vi "LSL with LVCS.vi"() -> ()   [LabVIEW 2016]
uses:
  source code/LSL components/output terminal/Plain OT/PainOutputTerminal.lvclass
  E:/Repository/LabVIEW Script Language/source code/LSL components/output terminal/Base/Output Terminal.lvclass
  source code/LSL components/scripts/scripts manager/scripts manager.lvclass
  source code/LSL components/variables/RT Variables/RT Variables.lvclass
  source code/LSL components/output terminal/Plain OT/PainOutputTerminal.lvclass/PainOutputTerminal.ctl
  <vilib>/ADI/Code String/Code String/Code String/Code String__adi.lvclass/Code String__adi.ctl
  source code/LSL components/scripts/scripts manager/scripts manager.lvclass/scripts manager.ctl
  source code/LSL components/scripts/scripts manager/properties/Write Scripts.vi
  source code/LSL components/output terminal/Plain OT/properties/Write Output Terminal.vi
  <vilib>/ADI/Code String/Code String/Code String LV/Code String LV__adi.lvclass
  C:/Program Files (x86)/National Instruments/LabVIEW 2016/vi.lib/ADI/Code String/Code String/Code String/Code String__adi.lvclass
  <vilib>/ADI/Code String/Code String/Code String LV/Create Code String LV.vi
  source code/LSL components/scripts/scripts manager/properties/Get Keywords.vi
  <vilib>/ADI/Code String/Code String/Code String/Properties/Write Keywords.vi
  <vilib>/ADI/Code String/Code String/Code String/Properties/Write Font Size.vi
  <vilib>/ADI/Code String/Code String/Code String/Properties/Write Completion.vi
  <vilib>/ADI/Code String/Code String/Code String/Properties/Write Delimiter Pattern.vi
  <vilib>/ADI/Code String/Code String/Code String/Properties/Write Editable.vi
  <vilib>/ADI/Code String/Code String/Code String/Properties/Write Text.vi
  <vilib>/ADI/Code String/Code String/Code String/Properties/Write Scroll Position.vi
  <vilib>/ADI/Code String/Code String/Code String/Properties/Write Selected Text.vi
  <vilib>/ADI/Code String/Code String/Code String/Properties/Write Font Color.vi
  <vilib>/ADI/Code String/Code String/Code String/Properties/Write Selection End.vi
  <vilib>/ADI/Code String/Code String/Code String/Properties/Write Selection Start.vi
  <vilib>/ADI/Code String/Code String/Code String/Properties/Read Selected Line(s).vi
  <vilib>/ADI/Code String/Code String/Code String/Properties/Read Selected Token.vi
  <vilib>/ADI/Code String/Code String/Code String/Properties/Read # Selected Lines.vi
  <vilib>/ADI/Code String/Code String/Code String/Properties/Read Selected Text.vi
  <vilib>/ADI/Code String/Code String/Code String/Properties/Read Text.vi
  <vilib>/ADI/Code String/Code String/Code String/Code String__adi.lvclass
panel:
  in  "Script Run":bool
  out "Output Terminal":string
  in  "Replacement Text":string="Test"
  in  "Replace Selection":bool
  out "Selected Text":string
  out "# Lines":i32
  out "Selected Token":string
  out "Selected Line(s)":string
  in  "Auto-complete":bool=TRUE
  in  "Editable":bool=TRUE
  in  "Checked?":bool
  out "Selected Menu Item":string
  in  "Item Name/Tag":string
  in  "Visible?":bool
  in  "Set Menu Item":bool
  in  "Selection End":u32
  in  "Selection Start":u32
  in  "Font Color":u32(colorbox)
  in  "Add Text":bool
  in  "Font Size":u32=14
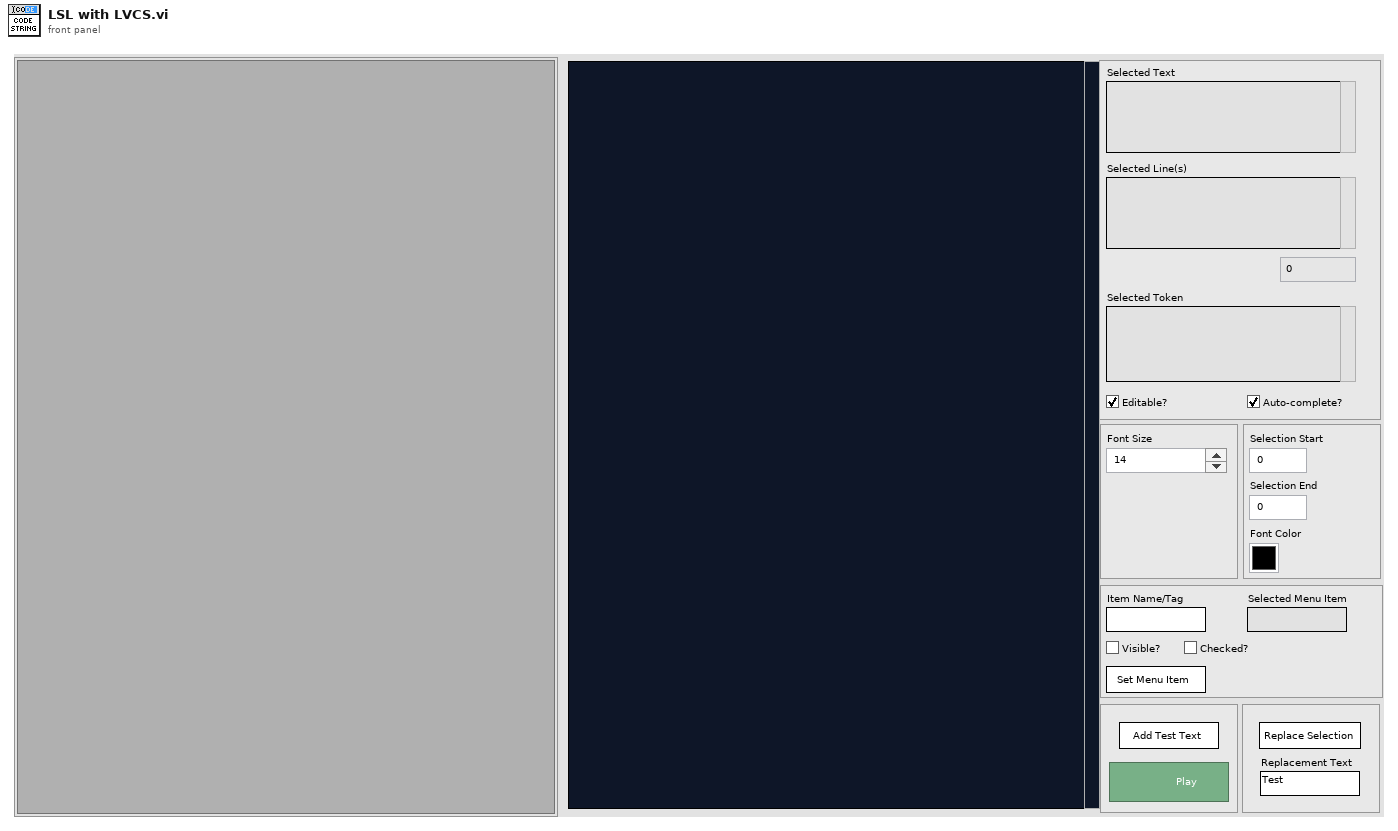
[diagram p1: front panel]
types:
  T1 = typedef "Code String__adi.lvclass/Public Events.ctl" = cluster{"Selected Token Changed":refnum<user-event>, "Value Changed":refnum<user-event>, "Shortcut Menu Selection":refnum<user-event>}
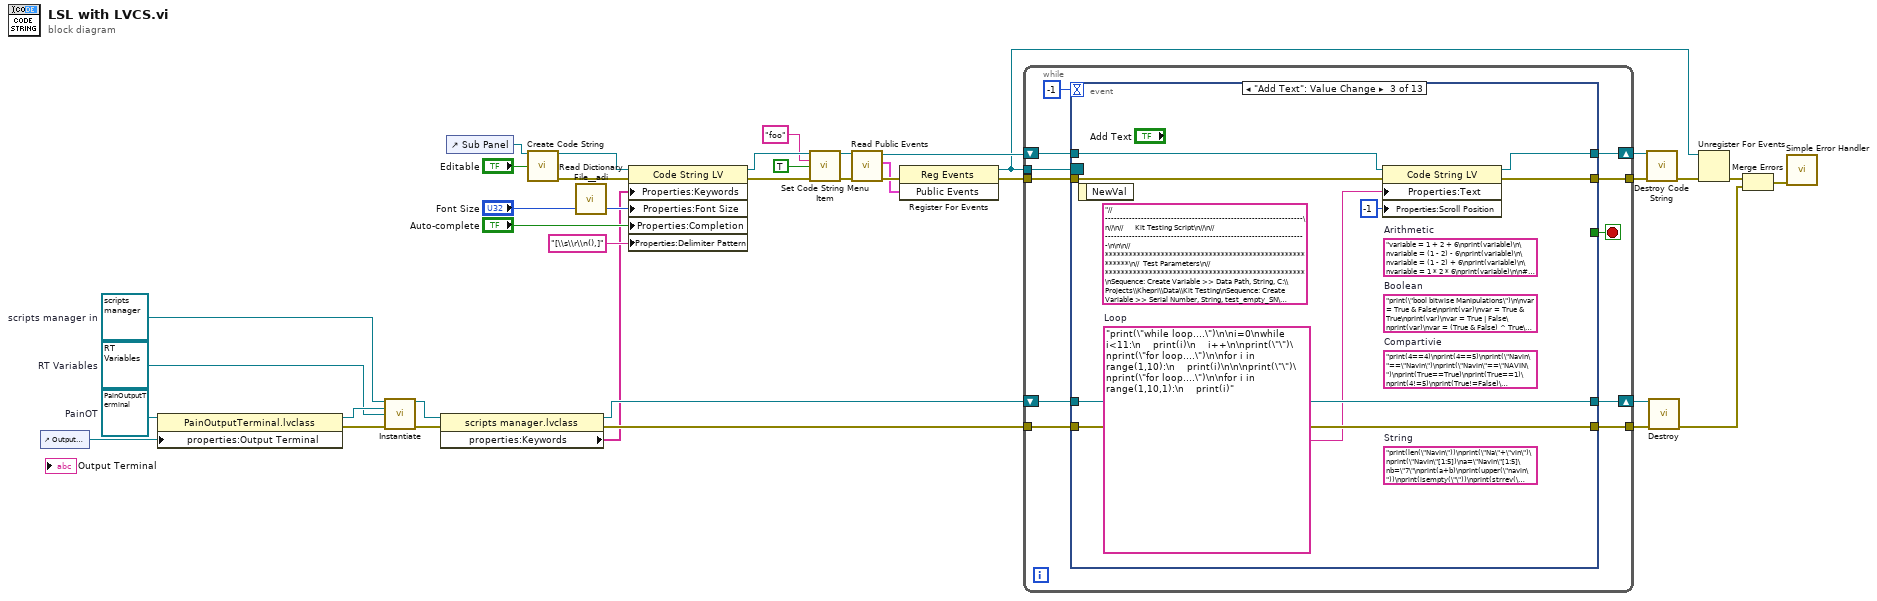
[diagram p0: block diagram]
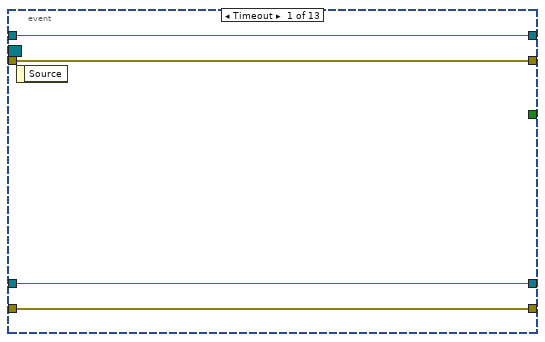
[diagram p2: hidden frame]
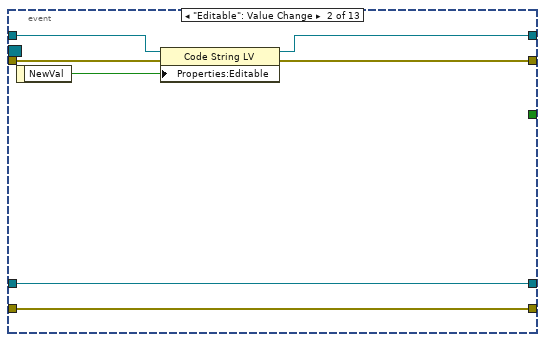
[diagram p3: hidden frame]
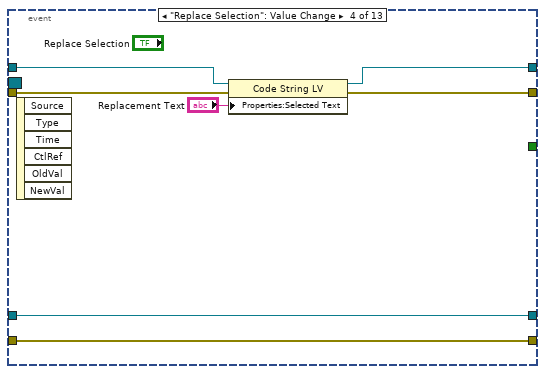
[diagram p4: hidden frame]
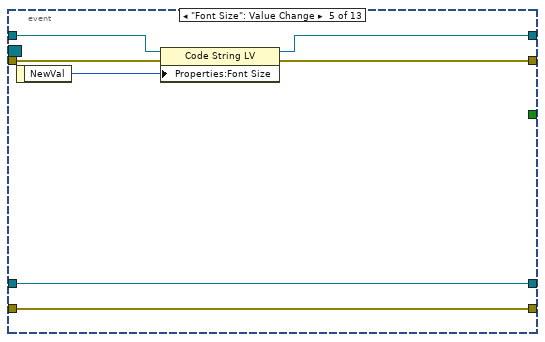
[diagram p5: hidden frame]
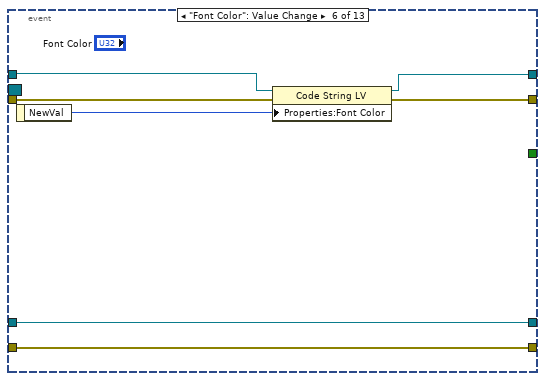
[diagram p6: hidden frame]
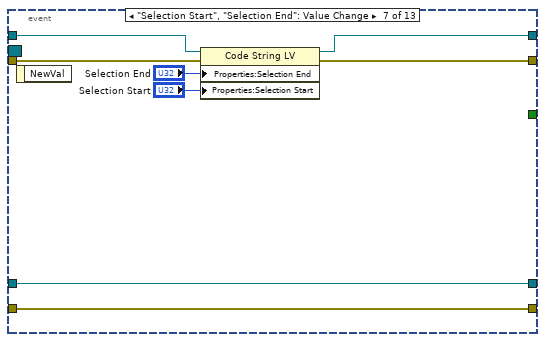
[diagram p7: hidden frame]
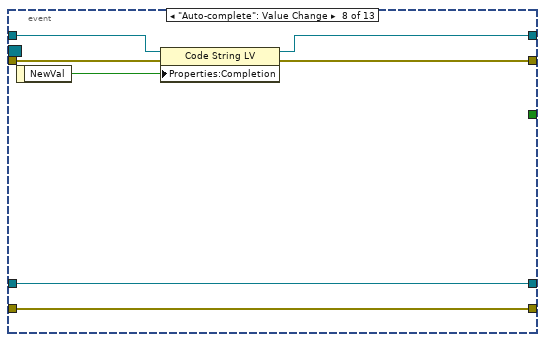
[diagram p8: hidden frame]
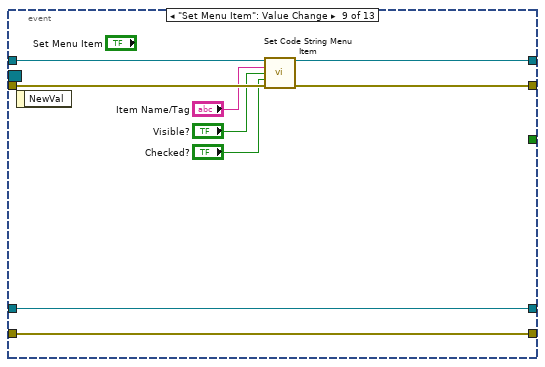
[diagram p9: hidden frame]
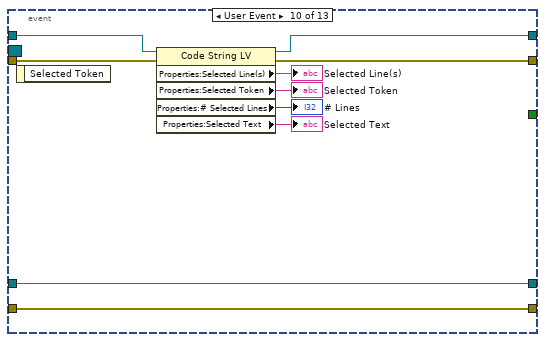
[diagram p10: hidden frame]
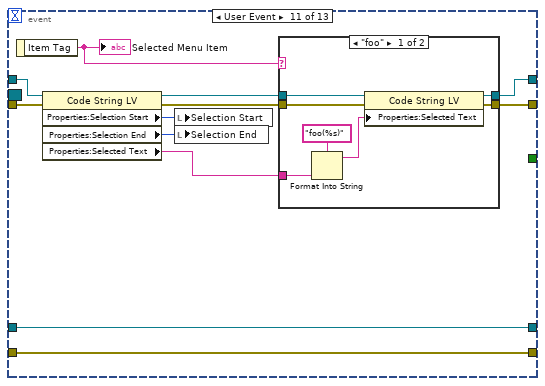
[diagram p11: hidden frame]
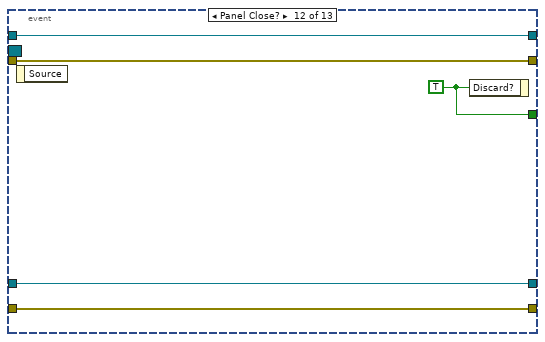
[diagram p13: hidden frame]
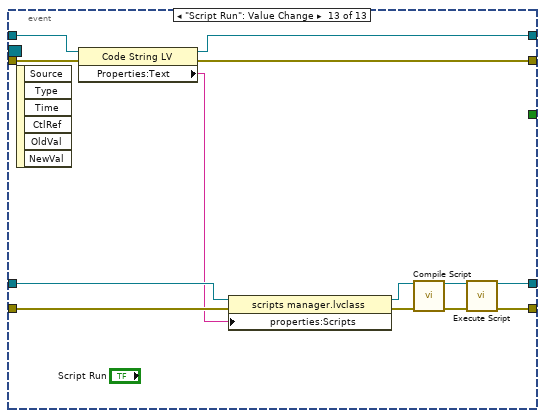
[diagram p14: hidden frame]
diagram:
  w10 = refnum<class "RT Variables.lvclass"> refnum  # RT Variables
  w12 = refnum<class "scripts manager.lvclass"> refnum  # scripts manager in
  w15 = refnum<class "PainOutputTerminal.lvclass"> refnum  # PainOT
  n1 = control-ref of="Output Terminal"() -> (w14:refnum<vi>)
  n2 = property class="PainOutputTerminal.lvclass"(reference=w15, "properties:Output Terminal"=w14) -> (reference out=w11:refnum<class "PainOutputTerminal.lvclass">, error out=w13:errorcluster)  [unwired: 1 in]
  n3 = call-dynamic "Instantiate.vi"("scripts manager in"=w12, "Output Terminal"=w11, "RT Variables"=w10, "error in (no error)"=w13) -> ("scripts manager out"=w3:refnum<class "scripts manager.lvclass">, "error out"=w9:errorcluster)  [unwired: 10 in]
  n4 = property class="scripts manager.lvclass"(reference=w3, error in=w9) -> (reference out=w2:refnum<class "scripts manager.lvclass">, error out=w4:errorcluster, "properties:Keywords"=w1:string[])
  n5 = control-ref of="Sub Panel"() -> (w21:refnum<vi>)
  n6 = call-poly <vilib>:"Create Code String.vi"("Subpanel"=w21, "Editable? (T)"="Editable") -> ("Code String LV"=w37:refnum<class "Code String LV__adi.lvclass">, "error out"=w33:errorcluster)  [unwired: 12 in]
  n7 = call "Read Dictionary File__adi.vi"() -> ()  [unwired: 3 in, 1 out]
  n8 = property class="Code String LV"(reference=w37, error in=w33, "Properties:Keywords"=w1, "Properties:Font Size"="Font Size", "Properties:Completion"="Auto-complete", "Properties:Delimiter Pattern"="[\\s\\r\\n(),]") -> (reference out=w19:refnum<class "Code String LV__adi.lvclass">, error out=w32:errorcluster)
  n9 = call <vilib>:"Set Code String Menu Item.vi"("Code String in"=w19, "Item Path"="foo", "Visibility (T)"=TRUE, "error in (no error)"=w32) -> ("Code String out"=w18:refnum<class "Code String LV__adi.lvclass">, "error out"=w20:errorcluster)  [unwired: 10 in]
  n10 = call <vilib>:"Read Public Events.vi"("error in (no error)"=w20, "Code String in"=w18) -> ("error out"=w29:errorcluster, "Public Events"=w26:T1, "Code String out"=w28:refnum<class "Code String LV__adi.lvclass">)  [unwired: 7 in]
  n11 = register-events(error in=w29, w26) -> (reference out=w23:refnum<event-registration>, error out=w27:errorcluster)  [unwired: 1 in]
  n12 = while {
    shift-right: [w47] -> w36
    shift-left: w28 -> [w48]
    tunnel: w27 -> [w46]
    tunnel: [w45] -> w35
    tunnel: w23 -> [w42]
    shift-right: [w39] -> w8
    shift-left: w2 -> [w41]
    tunnel: w4 -> [w40]
    tunnel: [w38] -> w7
    stop <- w43 stop-if-true
    n13 = event shown="[2] \"Add Text\": Value Change" {
      selector: w42 -> [_ _ _ _ _ _ _ _ _ _ _ _ _]
      dyn-events: _ -> [_ _ _ _ _ _ _ _ _ _ _ _ _]
      timeout: -1 -> [_ _ _ _ _ _ _ _ _ _ _ _ _]
      tunnel: w48 -> [w52 w58 w66 w72 w79 w84 w94 w101 w110 w120 w133 w146 w151]
      tunnel: [w52 w57 w65 w71 w78 w86 w93 w100 w109 w119 w126 w146 w150] -> w47
      tunnel: w46 -> [w51 w59 w67 w74 w81 w88 w96 w103 w112 w118 w134 w147 w153]
      tunnel: [w51 w56 w63 w73 w80 w87 w95 w102 w111 w117 w125 w147 w152] -> w45
      tunnel: [_ _ _ _ _ _ _ _ _ _ _ w148 _] -> w43
      tunnel: w41 -> [w50 w54 w62 w69 w76 w83 w90 w98 w105 w114 w124 w145 w159]
      tunnel: w40 -> [w49 w53 w61 w68 w75 w82 w89 w97 w104 w113 w123 w144 w161]
      tunnel: [w50 w54 w62 w69 w76 w83 w90 w98 w105 w114 w124 w145 w154] -> w39
      tunnel: [w49 w53 w61 w68 w75 w82 w89 w97 w104 w113 w123 w144 w155] -> w38
      event Timeout {
        n14 = event-data() -> ()  [unwired: 1 in, 1 out]
      }
      event "Editable": Value Change {
        n15 = event-data() -> ("NewVal"=w55:bool)  [unwired: 1 in]
        n16 = property class="Code String LV"(reference=w58, error in=w59, "Properties:Editable"=w55) -> (reference out=w57:refnum<class "Code String LV__adi.lvclass">, error out=w56:errorcluster)
      }
      event "Add Text": Value Change {
        (unwired) "print(len(\"Navin\"))\nprint(\"Na\"+\"vin\")\nprint(\"Navin\"[1:5])\na=\"Navin\"[1:5]\nb=\"7\"\nprint(a+b)\nprint(upper(\"navin\"))\nprint(isempty(\"\"))\nprint(strrev(\"navin\"))\n\na = \"Hello World!!!\"\nprint(a[1:6])\nprint(a[6])\n"  # String
        w60 = "print(\"while loop....\")\n\ni=0\nwhile i<11:\n    print(i)\n    i++\n\nprint(\"\")\nprint(\"for loop....\")\n\nfor i in range(1,10):\n    print(i)\n\n\nprint(\"\")\nprint(\"for loop....\")\n\nfor i in range(1,10,1):\n    print(i)"  # Loop
        (unwired) "print(4==4)\nprint(4==5)\nprint(\"Navin\"==\"Navin\")\nprint(\"Navin\"==\"NAVIN\")\nprint(True==True)\nprint(True==1)\nprint(4!=5)\nprint(True!=False)\nprint(1>2)\nprint(1<2)\nprint(1>=2)\nprint(1<=2)\n"  # Compartivie
        (unwired) "print(\"bool bitwise Manipulations\")\n\nvar = True & False\nprint(var)\nvar = True & True\nprint(var)\nvar = True | False\nprint(var)\nvar = (True & False) ^ True\nprint(var)\n\nprint(\"\")\nprint(\"numeric bitwise Manipulations\")\n\nvar1 = 1\nvar2 = 2\nprint(var1 & var2)\nprint(var1 | var2)\nprint(var1 ^ var2)\n\nprint(\"\")\nprint(\"bool Manipulations\")\n\nvar = True and False\nprint(var)\nvar = True and True\nprint(var)\nvar = True or False\nprint(var)\nvar = (True and False) xor True\nprint(var)\nprint(not(var))\n\nprint(\"\")\nprint(\"other functions\")\n\nprint(randombool())"  # Boolean
        (unwired) "variable = 1 + 2 + 6\nprint(variable)\n\nvariable = (1 - 2) - 6\nprint(variable)\n\nvariable = (1 - 2) + 6\nprint(variable)\n\nvariable = 1 * 2 * 6\nprint(variable)\n\n# a = gettick()\n\n#variable = (1 - 2) - (7-8) + (7/3.5) * 5 + (5+5) / 6 * 2 -1\nprint(variable)\n\n# print(\"time taken is : \"+str((gettick()-a)))\n\n# print(randomnumber())\n\n#the operation works from right to left\nvariable = (1 / 2 )/ 6\nprint(variable)\n\n#combination of operation\n\nvariable = 1 + 2 * 6 / 2\nprint(variable)\n\nvariable = 1 / 2 * 6 / 2\nprint(variable)\n\nvariable = 1 / 2 + 6 / 2\nprint(variable)\n\nvariable = ((1 / 2) - (6 * 2)) + 6.5\nprint(variable)\n\n# i=0\n# print(i++)\n# print(i--)\n\nvariable = ((1 - 2) - (6 * 2)) + 6.5\nprint(variable)\n\nvariable = 4%3\nprint(variable)\nprint(4%4)\nprint(4%5)\nprint(4%2)\n\nprint(4**2)\n\nprint(4//2)"  # Arithmetic
        (unwired) "//------------------------------------------------------------------\n//\n//      Kit Testing Script\n//\n//-------------------------------------------------------------------\n\n\n//********************************************************\n//  Test Parameters\n//**************************************************\nSequence: Create Variable >> Data Path, String, C:\\Projects\\Khepri\\Data\\Kit Testing\nSequence: Create Variable >> Serial Number, String, test_empty_SN\nSequence: Create Variable >> Noise Views, Integer, 512\n\nKit Testing: Scan Serial Number\nSequence: Update Variable >> Serial Number, = %Scanned Serial Number%\n\n//********************************************************\n// Sequence Variables\n//********************************************************\nSequence: Create Variable >> Gain, Integer, 0\nSequence: Create Variable >> Channel Counter, Integer, 0\n\n\n//Create a data folder for the serial number\nKit Testing: Create Folder >> %Data Path%\\%Serial Number%\nReports: Set Report Path >> %Data Path%\\%Serial Number%\n\n\nSequence: Library Call >> Board Control Library, Initialize Eval Boards\nDS: Write Value >> Eval_Register_Map/EvalRegMap:IO_CONTROL:IO_BGN_CTRL, = 0\nControl: Update Control Value >> View Rate, = 10\nControl: Update Control Value >> View Rate Slider, = 50\nControl: Update Control Value >> Set View Rate, = 1, Trigger\nSequence: Library Call >> Linearity Library, Clear 18bit Mode\n\n//%%%%%%%%%%%%%%%%%%%%%%%%%%%%%%%%%%%%%%%%%%%%%%%%%%\n//  Power Measurements\n//%%%%%%%%%%%%%%%%%%%%%%%%%%%%%%%%%%%%%%%%%%%%%%%%%%\n\nReports: New Datalog >> Voltage, Current\nPanels: Send Sync Command >> PXI-4113 - 1, 500, UI: Front Panel State >> Open\nPanels: Send Sync Command >> PXI-4113 - 2, 500, UI: Front Panel State >> Open\n\nPanels: Send Sync Command >>PXI-4113 - 1, 2000, Control: Update Control Value >> PXI 4113 Panel.CH0 Output, = 1, Trigger\nPanels: Send Sync Command >>PXI-4113 - 1, 2000, Control: Update Control Value >> PXI 4113 Panel.CH1 Output, = 1, Trigger\nPanels: Send Sync Command >>PXI-4113 - 2, 2000, Control: Update Control Value >> PXI 4113 Panel.CH1 Output, = 1, Trigger\nPanels: Send Sync Command >>PXI-4113 - 2, 2000, Control: Update Control Value >> PXI 4113 Panel.CH0 Output, = 1, Trigger\n\nUI: Generate Popup >> Move switch away from FPGA (LED off), then close shield\nDS: Write Value >> Eval_Register_Map/EvalRegMap:RELAYS_5:HB2, = 0\nFunction: Wait >> 0.1\nDS: Write Value >> Eval_Register_Map/EvalRegMap:RELAYS_5:HB2, = 1\nExperiments: Program FPGA >> C:\\Projects\\Khepri\\Labview\\Firmware\\Sphinx\\sphinx_320ADC_DBG_051818.bin\n\n//Wait 5 seconds for the DUT board to initialize and program\nFunction: Wait >> 5\n\nPanels: Send Sync Command >>PXI-4113 - 1, 2000, Control: Update Control Value >> PXI 4113 Panel.Measure Supplies, = 1, Trigger\nPanels: Send Sync Command >>PXI-4113 - 2, 2000, Control: Update Control Value >> PXI 4113 Panel.Measure Supplies, = 1, Trigger\n\nReports: Datalog >> %PXI-4113 - 1: PXI 4113 Panel.CH0 Voltage%, %PXI-4113 - 1: PXI 4113 Panel.CH0 Current%, M{%PXI-4113 - 1: PXI 4113 Panel.CH0 Voltage% * %PXI-4113 - 1: PXI 4113 Panel.CH0 Current%}, W, Fractional, Total Power\nReports: Datalog >> %PXI-4113 - 1: PXI 4113 Panel.CH1 Voltage%, %PXI-4113 - 1: PXI 4113 Panel.CH1 Current%, M{%PXI-4113 - 1: PXI 4113 Panel.CH1 Voltage% * %PXI-4113 - 1: PXI 4113 Panel.CH1 Current%}, W, Fractional, Total Power\nReports: Datalog >> %PXI-4113 - 2: PXI 4113 Panel.CH0 Voltage%, %PXI-4113 - 2: PXI 4113 Panel.CH0 Current%, M{%PXI-4113 - 2: PXI 4113 Panel.CH0 Voltage% * %PXI-4113 - 2: PXI 4113 Panel.CH0 Current%}, W, Fractional, Total Power\nReports: Datalog >> %PXI-4113 - 2: PXI 4113 Panel.CH1 Voltage%, %PXI-4113 - 2: PXI 4113 Panel.CH1 Current%, M{%PXI-4113 - 2: PXI 4113 Panel.CH1 Voltage% * %PXI-4113 - 2: PXI 4113 Panel.CH1 Current%}, W, Fractional, Total Power \n\nReports: Set Report Name >> %Serial Number%_Power\nReports: Save Datalog >> Close\n\nPanels: Send Sync Command >> PXI-4113 - 1, 500, UI: Front Panel State >> Close\nPanels: Send Sync Command >> PXI-4113 - 2, 500, UI: Front Panel State >> Close\n\n\n//+++++++++++++++++++++++++++++++++++++++++++++++++++++++++++++++++\n//  Noise and Offset tests\n//+++++++++++++++++++++++++++++++++++++++++++++++++++++++++++++++++\nReports: New Report\n\nControl: Update Control Value >> Eval Tabs, = 0\nReports: New Datalog >> View Rate, VR Jitter, Gain, Max Offset, Min Offset, Max Noise, Mean Noise\n\n//Connect Q_BOARD_AGND_PDA to BOARD_DGND\nSequence: Library Call >> Board Control Library, Power Up Slave Eval\nSequence: Library Call >> Noise and Offset Library, Set Noise Master Relays\n//Sequence: Library Call >> Board Control Library, Power Down Slave Eval\nSequence: Call >> Initialize Noise Test Parameters\n\n\n\n//Set View rate to 3000min\nControl: Update Control Value >> View Rate, = 10\nControl: Update Control Value >> View Rate Slider, = 0\nControl: Update Control Value >> Set View Rate, = 1, Trigger\n\n//Run Noise and Offset versus gain setting\nSequence: Call >> Noise and Offset versus Gain\n\n//Set View rate to 800max\nControl: Update Control Value >> View Rate, = 0\nControl: Update Control Value >> View Rate Slider, = 100\nControl: Update Control Value >> Set View Rate, = 1, Trigger\n\n//Run Noise and Offset versus gain setting\nSequence: Call >> Noise and Offset versus Gain\n\n//Set View rate to 3000nom\nControl: Update Control Value >> View Rate, = 10\nControl: Update Control Value >> View Rate Slider, = 50\nControl: Update Control Value >> Set View Rate, = 1, Trigger\n\nReports: Set Report Name >> %Serial Number%_Noise_and_Offset\nReports: Save Datalog >> Close\n\nSequence: Library Call >> Board Control Library, Power Up Slave Eval\nSequence: Library Call >> Noise and Offset Library, Clear Noise Master Relays\n\n\n//End Noise and Offset Tests\n//+++++++++++++++++++++++++++++++++++++++++++++++++++++++++++++\n\n\n//====================================================\n//  Linearity Tests\n//====================================================\n\nReports: New Line\nControl: Update Control Value >> Eval Tabs, = 1\n\nSequence: Library Call >> Board Control Library, Power Up Slave Eval\n\nSequence: Library Call >> Board Control Library, Power Up Master Q Board\nSequence: Library Call >> Board Control Library, Power Up Slave Q Board\nFunction: Wait >> 3\n\n//Set the Analog Input Relays to connect Q board to DUT\nPanels: Send Sync Command >>Khepri Panel, 8000, Control: Update Control Value >> Set Master Analog Relays, = 1, Trigger\nPanels: Send Sync Command >>Khepri Panel, 8000, Control: Update Control Value >> Set Slave Analog Relays, = 1, Trigger\n\nSequence: Library Call >> Linearity Library, Default Linearity Processing Settings\n\n\nSequence: Library Call >> Linearity Library, Set 18bit Mode\n\n\n\nSequence: For >> Gain = 1; Gain <= 7; Gain + 1\nReports: New Datalog >> Gain, Max INL, Max INL CH, Min INL, Min INL CH, Max Gain, Max Gain CH, Min Gain, Min Gain CH\n\nDS: Write Value >> Eval_Register_Map/EvalRegMap:TRS_HEADER_DAT:GAIN, = %Gain%\nSequence: Library Call >> Linearity Library, Linearity Gain%Gain% Settings\nControl: Update Control Value >> Run Linearity, = T, Trigger\nReports: Add Comment >> Gain %Gain% Linearity\nReports: Add Picture >> Linearity\nReports: Add Picture >> Raw Data\nReports: New Page\n\nReports: Datalog >> %Gain%, %Linearity Results.Max INL%, %Linearity Results.Max INL CH%, %Linearity Results.Min INL%, %Linearity Results.Min INL CH%, %Linearity Results.Max Gain%, %Linearity Results.Max Gain CH%, %Linearity Results.Min Gain%, %Linearity Results.Min Gain CH%, 0, Linearity, Fractional, All the linearity datas\n\n\nReports: Datalog Array >> Gain per Channel, Gain per channel\nReports: Datalog Array >> DAC Input Values, Linearity Input Values\n\nSequence: For >> Channel Counter = 0; Channel Counter <= 191; Channel Counter + 1\nKit Testing: Get Linearity Ain Data >> %Channel Counter%\nReports: Datalog Array >> CH%Channel Counter% Linearity, Linearity Ain Data\nSequence: END FOR\n\nReports: Set Report Name >> %Serial Number%_G%Gain%_Linearity_and_Gain\nReports: Save Datalog >> Close\n\nSequence: END FOR\n\n\n//Open Analog Input relays again\nPanels: Send Sync Command >>Khepri Panel, 8000, Control: Update Control Value >> Reset Master Analog Relays, = 1, Trigger\nPanels: Send Sync Command >>Khepri Panel, 8000, Control: Update Control Value >> Reset Slave Analog Relays, = 1, Trigger\n\nSequence: Library Call >> Linearity Library, Clear 18bit Mode\nSequence: Library Call >> Board Control Library, Power Down Slave Q Board\nSequence: Library Call >> Board Control Library, Power Down Master Q Board\nSequence: Library Call >> Board Control Library, Power Down Slave Eval\n\n\n//End Linearity Tests\n//====================================================================\n\n\n\n//#############################################################################\n//  Input Leakage and Offset Drift\n//#############################################################################\nControl: Update Control Value >> Eval Tabs, = 4\nControl: Update Control Value >> Tests Subtabs, = 3\n\n\nReports: New Datalog >> Offset Drift\n\n//Offset drift settings\nControl: Update Control Value >> Total Time (sec), = 65\nControl: Update Control Value >> Moving Average Window, = 144\nDS: Write Value >> Eval_Register_Map/EvalRegMap:TRS_HEADER_DAT:GAIN, = 3\nDS: Write Value >> Eval_Register_Map/EvalRegMap:NUM_VIEWS_CAPT:NUM_VIEWS_CAPT, = 256\nControl: Update Control Value >> View Rate Slider, = 50\nControl: Update Control Value >> View Rate, = 10\nControl: Update Control Value >> Set View Rate, = 1, Trigger\nControl: Update Control Value >> Offset Drift Processing.Display, = 0\n\nControl: Update Control Value >> Run Offset Drift, = 1, Trigger\n\nReports: Add Picture >> Offset Drift Graph\nReports: Datalog Array >> Offset Drift, Drift Data per Channel\nReports: Set Report Name >> %Serial Number%_G3_Offset_Drift\nReports: Save Datalog >> Close\nFunction: Wait >> 2\n\n\n//This is the recorded macro sequence\n***\nReports: New Datalog >> Input Leakage\n\n//Input Leakage settings\nControl: Update Control Value >> First Edge Clock, = 775\nControl: Update Control Value >> Start Clock, = 5000\nControl: Update Control Value >> End Clock, = 12000\nControl: Update Control Value >> Num Leakage Steps, = 10\nDS: Write Value >> Eval_Register_Map/EvalRegMap:TRS_HEADER_DAT:GAIN, = 1\nDS: Write Value >> Eval_Register_Map/EvalRegMap:NUM_VIEWS_CAPT:NUM_VIEWS_CAPT, = 64\nDS: Write Value >> Eval_Register_Map/EvalRegMap:VT_LOW_BITS:VT_PERIOD, = 1000000\n\nControl: Update Control Value >> Run Input Leakage, = 1, Trigger\n\n\nReports: Datalog Array >> Input Leakage, Leakage Data per Channel\nReports: Set Report Name >> %Serial Number%_G1_Input_Leakage\nReports: Save Datalog >> Close\n***\n\nReports: Set Report Name >> %Serial Number%_Results\nReports: Save Report >> Close\n\n\nUI: Generate Popup >> Move switch toward FPGA (LED on)\nExperiments: Program EEPROM >> C:\\Projects\\Khepri\\Labview\\Firmware\\Sphinx\\sphinx_320ADC_DBG_051818.bin\n\n//Power down the board at the end of the sequence\nPanels: Send Sync Command >>PXI-4113 - 2, 2000, Control: Update Control Value >> PXI 4113 Panel.CH0 Output, = 0, Trigger\nPanels: Send Sync Command >>PXI-4113 - 2, 2000, Control: Update Control Value >> PXI 4113 Panel.CH1 Output, = 0, Trigger\nPanels: Send Sync Command >>PXI-4113 - 1, 2000, Control: Update Control Value >> PXI 4113 Panel.CH0 Output, = 0, Trigger\nPanels: Send Sync Command >>PXI-4113 - 1, 2000, Control: Update Control Value >> PXI 4113 Panel.CH1 Output, = 0, Trigger\n\nSequence: END SEQUENCE\n\nSequence: Subroutine >> Initialize Noise Test Parameters\n//Initialize Noise Test\nDS: Write Value >> Eval_Register_Map/EvalRegMap:TRS_HEADER_DAT:GAIN, = 0\nDS: Write Value >> Eval_Register_Map/EvalRegMap:IO_CONTROL:IO_BGN_CTRL, = 0\nDS: Write Value >> Eval_Register_Map/EvalRegMap:NUM_VIEWS_CAPT:NUM_VIEWS_CAPT, = %Noise Views%\nControl: Update Control Value >> Data Display, = 4, Trigger\nSequence: Return\n\n\n\nSequence: Subroutine >> Noise and Offset versus Gain\n//Your Subroutine code here\nSequence: For >> Gain = 0; Gain <= 7; Gain + 1\nDS: Write Value >> Eval_Register_Map/EvalRegMap:TRS_HEADER_DAT:GAIN, = %Gain%\nFunction: Wait >> 0.100000\nControl: Update Control Value >> Single Capture, = 1, Trigger\n\nReports: Datalog Array >> %View Rate Value% G%Gain% Offset, Pixel Data.Mean per pixel\nReports: Datalog Array >> %View Rate Value% G%Gain% Noise, Pixel Data.Noise per pixel\nReports: Datalog >> %View Rate Value%, %View Rate Slider%, %Gain%, %Pixel Data.Max Offset%, %Pixel Data.Min Offset%, %Pixel Data.Max Noise%, %Pixel Data.Mean Noise%, 0, LSBs, Fractional, All the data\n\nReports: Add Comment >> Gain%Gain% - %View Rate Value%vps\nReports: Add Picture >> Waveform\nSequence: END FOR\nSequence: Return\n"
        n17 = event-data() -> ()  [unwired: 1 in, 1 out]
        n18 = property class="Code String LV"(reference=w66, error in=w67, "Properties:Text"=w60, "Properties:Scroll Position"=-1) -> (reference out=w65:refnum<class "Code String LV__adi.lvclass">, error out=w63:errorcluster)
      }
      event "Replace Selection": Value Change {
        n19 = event-data() -> ()  [unwired: 1 in, 6 out]
        n20 = property class="Code String LV"(reference=w72, error in=w74, "Properties:Selected Text"="Replacement Text") -> (reference out=w71:refnum<class "Code String LV__adi.lvclass">, error out=w73:errorcluster)
      }
      event "Font Size": Value Change {
        n21 = event-data() -> ("NewVal"=w77:u32)  [unwired: 1 in]
        n22 = property class="Code String LV"(reference=w79, error in=w81, "Properties:Font Size"=w77) -> (reference out=w78:refnum<class "Code String LV__adi.lvclass">, error out=w80:errorcluster)
      }
      event "Font Color": Value Change {
        n23 = event-data() -> ("NewVal"=w85:u32)  [unwired: 1 in]
        n24 = property class="Code String LV"(reference=w84, error in=w88, "Properties:Font Color"=w85) -> (reference out=w86:refnum<class "Code String LV__adi.lvclass">, error out=w87:errorcluster)
      }
      event "Selection Start", "Selection End": Value Change {
        n25 = event-data() -> ()  [unwired: 1 in, 1 out]
        n26 = property class="Code String LV"(reference=w94, error in=w96, "Properties:Selection End"="Selection End", "Properties:Selection Start"="Selection Start") -> (reference out=w93:refnum<class "Code String LV__adi.lvclass">, error out=w95:errorcluster)
      }
      event "Auto-complete": Value Change {
        n27 = event-data() -> ("NewVal"=w99:bool)  [unwired: 1 in]
        n28 = property class="Code String LV"(reference=w101, error in=w103, "Properties:Completion"=w99) -> (reference out=w100:refnum<class "Code String LV__adi.lvclass">, error out=w102:errorcluster)
      }
      event "Set Menu Item": Value Change {
        n29 = event-data() -> ()  [unwired: 1 in, 1 out]
        n30 = call <vilib>:"Set Code String Menu Item.vi"("Code String in"=w110, "Item Path"="Item Name/Tag", "Visibility (T)"="Visible?", "Checked (F)"="Checked?", "error in (no error)"=w112) -> ("Code String out"=w109:refnum<class "Code String LV__adi.lvclass">, "error out"=w111:errorcluster)  [unwired: 9 in]
      }
      event User Event {
        n31 = event-data() -> ()  [unwired: 1 in, 1 out]
        n32 = property class="Code String LV"(reference=w120, error in=w118) -> (reference out=w119:refnum<class "Code String LV__adi.lvclass">, error out=w117:errorcluster, "Properties:Selected Line(s)"=→"Selected Line(s)":string, "Properties:Selected Token"=→"Selected Token":string, "Properties:# Selected Lines"=→"# Lines":i32, "Properties:Selected Text"=→"Selected Text":string)
      }
      event User Event {
        n33 = event-data() -> ("Item Tag"=w130:string)  [unwired: 1 in]
        "Selected Menu Item" <- w130
        n34 = property class="Code String LV"(reference=w133, error in=w134) -> (reference out=w127:refnum<class "Code String LV__adi.lvclass">, error out=w128:errorcluster, "Properties:Selection Start"=w131:u32, "Properties:Selection End"=w132:u32, "Properties:Selected Text"=w129:string)
        n35 = local write "Selection Start"(w131) -> ()
        n36 = local write "Selection End"(w132) -> ()
        n37 = case shown="\"foo\"" w130 {
          tunnel: w129 -> [w141 _]
          tunnel: w128 -> [w139 w143]
          tunnel: w127 -> [w138 w142]
          tunnel: [w137 w142] -> w126
          tunnel: [w135 w143] -> w125
          frame "foo" {
            n38 = Format Into String(format string="foo(%s)", w141) -> (resulting string=w136:string)  [unwired: 2 in, 1 out]
            n39 = property class="Code String LV"(reference=w138, error in=w139, "Properties:Selected Text"=w136) -> (reference out=w137:refnum<class "Code String LV__adi.lvclass">, error out=w135:errorcluster)
          }
          frame Default {
          }
        }
      }
      event Panel Close? {
        w148 = TRUE ("Discard?")
        n40 = event-data() -> ()  [unwired: 1 in, 1 out]
        n41 = event-data("Discard?"=w148) -> ()  [unwired: 1 in, 1 out]
      }
      event "Script Run": Value Change {
        n42 = event-data() -> ()  [unwired: 1 in, 6 out]
        n43 = property class="Code String LV"(reference=w151, error in=w153) -> (reference out=w150:refnum<class "Code String LV__adi.lvclass">, error out=w152:errorcluster, "Properties:Text"=w149:string)
        n44 = property class="scripts manager.lvclass"(reference=w159, error in=w161, "properties:Scripts"=w149) -> (reference out=w158:refnum<class "scripts manager.lvclass">, error out=w160:errorcluster)
        n45 = call-dynamic "Compile Script.vi"("scripts manager in"=w158, "error in (no error)"=w160) -> ("scripts manager out"=w156:refnum<class "scripts manager.lvclass">, "error out"=w157:errorcluster)  [unwired: 12 in]
        n46 = call-dynamic "Execute Script.vi"("scripts manager in"=w156, "error in (no error)"=w157) -> ("scripts manager out"=w154:refnum<class "scripts manager.lvclass">, "error out"=w155:errorcluster)  [unwired: 12 in]
      }
    }
  }
  n47 = call <vilib>:"Destroy Code String.vi"("Code String in"=w36, "error in (no error)"=w35) -> ("error out"=w34:errorcluster)  [unwired: 12 in, 1 out]
  n48 = call-dynamic "Destroy.vi"("scripts manager in"=w8, "error in (no error)"=w7) -> ("error out"=w5:errorcluster)  [unwired: 12 in, 1 out]
  n49 = Unregister For Events(event registration refnum=w23, error in=w34) -> (error out=w24:errorcluster)
  n50 = Merge Errors(w24, w5) -> (w6:errorcluster)
  n51 = call <vilib>:"Simple Error Handler.vi"("error in (no error)"=w6) -> ()  [unwired: 4 in, 5 out]
